vi "Fetch Room Details.vi"(0 "Rooms Manager Model in":refnum<class "Rooms Manager Model.lvclass">, 5 "Room No":string, 11 "error in (no error)":errorcluster) -> (4 "Rooms Manager Model out":refnum<class "Rooms Manager Model.lvclass">, 15 "error out":errorcluster)   [LabVIEW 2023, in "Rooms Manager Model.lvlib" / "Rooms Manager Model.lvclass"]
uses:
  Rooms Manager Model.lvclass
  Rooms Manager Model.lvclass/Rooms Manager Model.ctl
  <vilib>/ActorFramework/Actor/Actor.lvclass
  Interfaces/Incoming Hotel Management Tool Model Interface Messages/Fetch Room Details Msg/Fetch Room Details Msg.lvclass
  C:/Users/bhaghyaraj/Trainings/NI Actor Framework/SDLC/Model Base/Model Base/Model Base.lvclass
  C:/Program Files/National Instruments/LabVIEW 2023/vi.lib/ActorFramework/Actor/Actor.lvclass
  C:/Users/bhaghyaraj/Trainings/NI Actor Framework/SDLC/Interfaces/Model Base/Incoming Model Base Interface.lvclass
  C:/Users/bhaghyaraj/Trainings/NI Actor Framework/SDLC/Rooms Manager Model/Rooms Manager Model/Rooms Manager Model.lvclass
  C:/Users/bhaghyaraj/Trainings/NI Actor Framework/SDLC/Interfaces/Rooms Manager Model/Incoming Rooms Manager Model Interface.lvclass
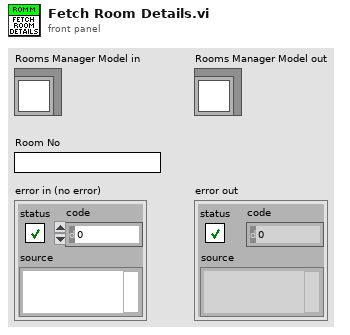
[diagram p1: front panel]
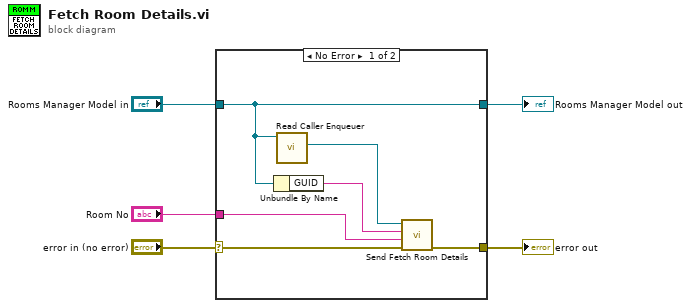
[diagram p0: block diagram]
diagram:
  n1 = case shown="No Error" "error in (no error)" {
    selector: "error in (no error)" -> [w11 w12]
    tunnel: [w10 w12] -> w2
    tunnel: "Room No" -> [w6 _]
    tunnel: "Rooms Manager Model in" -> [w8 w13]
    tunnel: [w8 w13] -> w5
    frame No Error {
      n2 = Unbundle By Name(w8) -> ("GUID"=w7:string)
      n3 = call <vilib>:"Read Caller Enqueuer.vi"("Actor"=w8) -> ("Caller Enqueuer"=w9:refnum<class "Message Enqueuer.lvclass">)  [unwired: 10 in]
      n4 = call "Send Fetch Room Details.vi"("error in (no error)"=w11, "Room No"=w6, "Rooms Manager GUID"=w7, "Message Enqueuer"=w9) -> ("error out"=w10:errorcluster)  [unwired: 6 in, 1 out]
    }
    frame Error {
    }
  }
  "error out" <- w2
  "Rooms Manager Model out" <- w5
